vi "Proyecto Autotronicacopyy.vi"() -> ()   [LabVIEW 2026]
uses:
  <vilib>/MakerHub/LINX/Private/Type Defs/LINX Ref.ctl
  <vilib>/MakerHub/LINX/Private/Type Defs/Platform.ctl
  <vilib>/MakerHub/LINX/Private/Type Defs/Interface.ctl
  <vilib>/MakerHub/LINX/Private/Device/Type Defs/LINX Device Config.ctl
  <vilib>/MakerHub/LINX/Private/Device/Type Defs/TCP Config.ctl
  <vilib>/MakerHub/LINX/Private/Device/Type Defs/Channels.ctl
  <vilib>/MakerHub/LINX/Public/Peripherals/Digital/Digital Read 1 Chan.vi
  <vilib>/MakerHub/LINX/Public/Peripherals/Analog/Analog Read 1 Chan.vi
  <vilib>/MakerHub/LINX/Public/Peripherals/Digital/Digital Read N Chans.vi
  <vilib>/MakerHub/LINX/Public/Peripherals/Analog/Analog Read N Chans.vi
  <vilib>/MakerHub/LINX/Private/Local IO/LinxDigitalRead.vi
  <vilib>/MakerHub/LINX/Public/Utilities/Check Channel.vi
  <vilib>/MakerHub/LINX/Private/Local IO/LinxAnalogRead.vi
  <vilib>/MakerHub/LINX/Public/Utilities/Open Serial.vi
  <vilib>/MakerHub/LINX/Private/Utilties/Generate Error.vi
  <vilib>/express/express shared/transition.llb/Dynamic To Waveform Array.vi
  <vilib>/express/express signal manip/GetorSetDDTAttributes/Set DDT Attributes/SetT0.vi
  <vilib>/express/express signal manip/GetorSetDDTAttributes/Set DDT Attributes/sub Set StartTimeStamp.vi
  <vilib>/express/express shared/transition.llb/Waveform Array To Dynamic.vi
  <vilib>/express/express signal manip/GetorSetDDTAttributes/Set DDT Attributes/Set DDT Properties.xnode
  <vilib>/express/express arith-compare/Formula/XNode/ExpressFormulaBlockNode.xnode
  <vilib>/MakerHub/LINX/LMH-LINX.lvlib
  <vilib>/MakerHub/LINX/Private/Device/Device.lvlib
  <vilib>/express/express signal manip/GetorSetDDTAttributes/Set DDT Attributes/Set DDT Attributes.lvlib
panel:
  out "Waveform Chart":dbl(graph)
  out "BAR":dbl format="%#_3g"
  out "Km/hora":dbl format="%#.2g"
  out "TRAS_DER 4":bool
  out "TRAS_IZQ 3":bool
  out "DEL_IZQ":bool
  out "DEL:DER  2":bool
  out "Millas/hora":dbl format="%#.2g"
  out "Puerta 2":bool
  out "Puerta 3":bool
  out "Puerta 1":bool
  out "Llanta trasera/der":u8(slide) scale=0.0..40.0
  out "PSI":dbl format="%#_3g"
  out "BAR 2":dbl format="%#_2g"
  out "Llanta trasera/der  2":dbl(knob) scale=0.0..40.0
  out "Llanta trasera/izq":u8(slide) scale=0.0..40.0
  out "Gauge":dbl(knob) scale=0.0..200.0
  out "PSI 2":dbl format="%#_4g"
  out "BAR 3":dbl format="%#_3g"
  out "Llanta trasera/izq  2":dbl(knob) scale=0.0..40.0
  out "Llanta delantera/der":u8(slide) scale=0.0..40.0
  out "PSI 3":dbl format="%#_4g"
  out "BAR 4":dbl caption="BAR" format="%#_3g"
  out "Llanta delantera/der  2":dbl(knob) scale=0.0..40.0
  out "Llanta delantera/izq":u8(slide) scale=0.0..40.0
  out "PSI 4":dbl format="%#_4g"
  out "Llanta delantera/izq 2":dbl(knob) scale=0.0..40.0
  in  "stop":bool
  in  "Serial Port":refnum<visa-resource-name>="N/A"
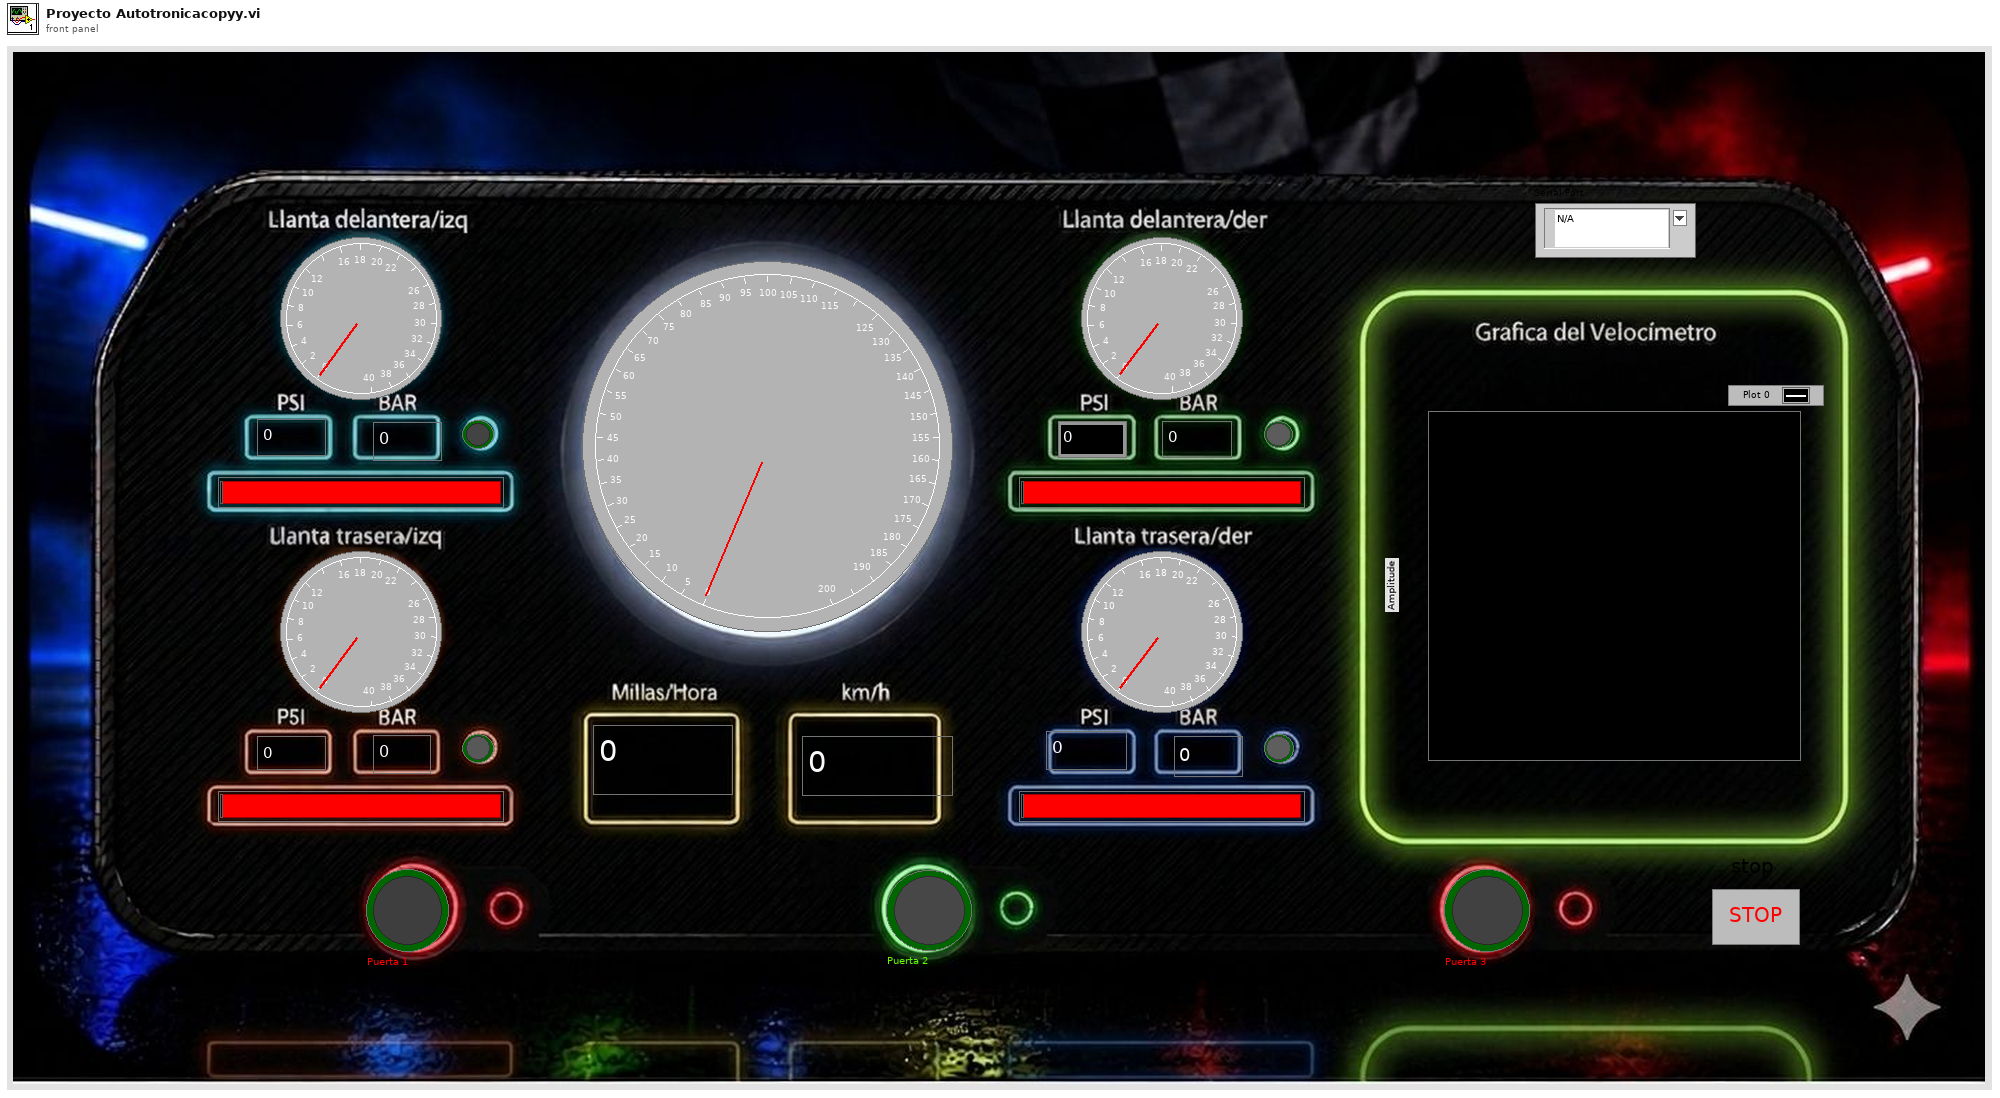
[diagram p1: front panel]
types:
  T1 = typedef "LMH-LINX.lvlib/LINX Ref.ctl" = cluster{"IO":T2, "Interface":T3, "LINX Device Config":T4}
  T2 = typedef "LMH-LINX.lvlib/Platform.ctl" = enum16{"Remote", "Local"}
  T3 = typedef "LMH-LINX.lvlib/Interface.ctl" = enum16{"Serial", "TCP"}
  T4 = typedef "LMH-LINX.lvlib/Device.lvlib/LINX Device Config.ctl" = cluster{"Interface":T3, "COM Port":refnum<visa-resource-name>, "TCP Configuration":T5, "Device Family":u8, "Device ID":u8, "Device Name":string, "TCP Ref":refnum<k5>, "Channels":T6}
  T5 = typedef "LMH-LINX.lvlib/Device.lvlib/TCP Config.ctl" = cluster{"IP Address":string, "Port":u16}
  T6 = typedef "LMH-LINX.lvlib/Channels.ctl" = cluster{"DI":u8[], "DO":u8[], "AI":u8[], "AO":u8[], "PWM":u8[], "QE":u8[], "UART":u8[], "I2C 2":u8[], "SPI":u8[], "CAN":u8[], "Servo":u8[], "AI Ref (V)":dbl, "AI Resolution (Bits)":u8, "AO Ref (V)":dbl, "AO Resolution (Bits)":u8}
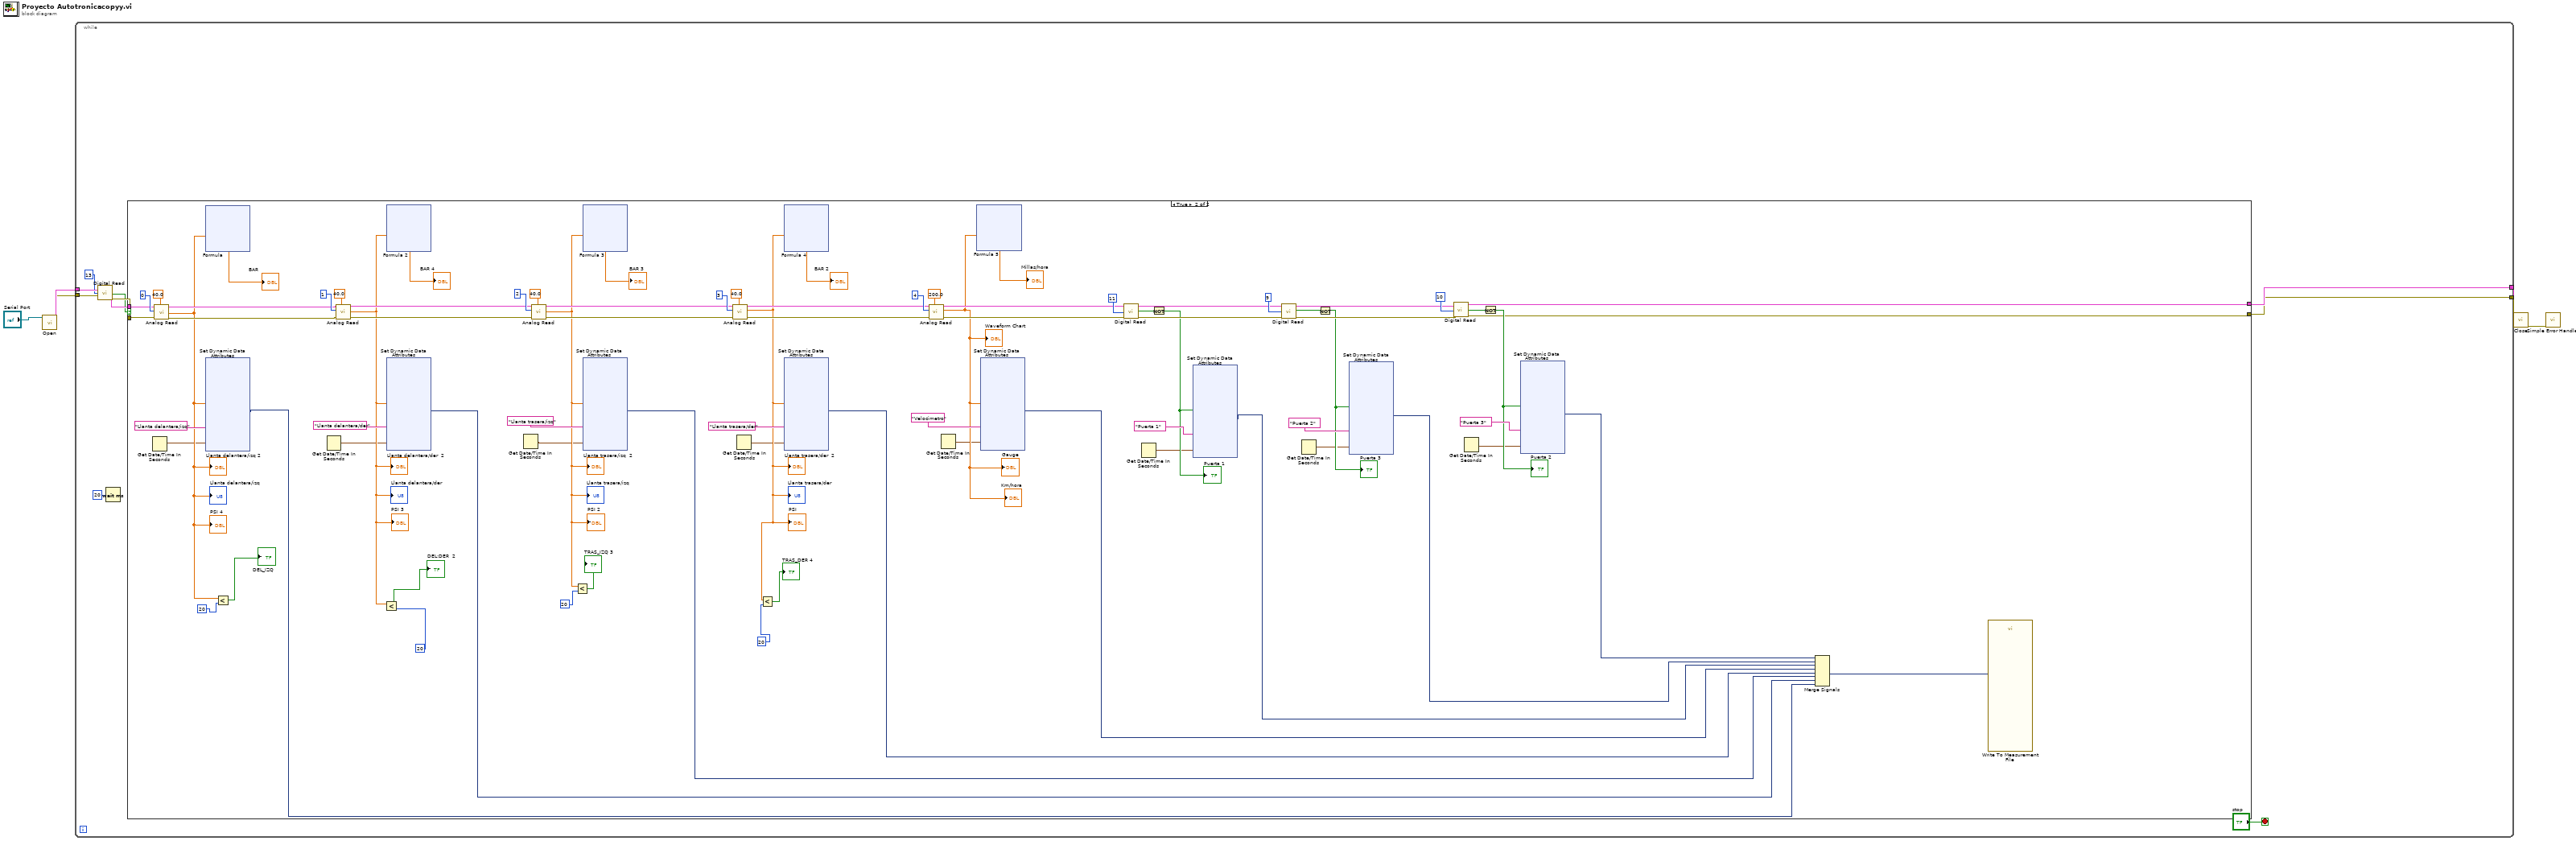
[diagram p0: block diagram]
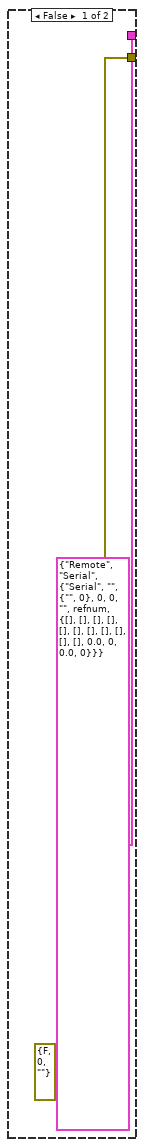
[diagram p2: hidden frame]
diagram:
  n1 = call-poly <vilib>:"Open.vi"("Serial Port"="Serial Port") -> ("Error Out"=w4:errorcluster, "LINX Resource"=w5:T1)  [unwired: 8 in, 1 out]
  n2 = while {
    tunnel: w5 -> [w16]
    tunnel: w4 -> [w15]
    tunnel: [w10] -> w1
    tunnel: [w9] -> w2
    stop <- "stop" stop-if-true
    n3 = call-poly <vilib>:"Digital Read.vi"("Error In"=w15, "DI Channel"=13, "LINX Resource"=w16) -> ("Error Out"=w12:errorcluster, "DI Value"=w7:bool, "LINX Resource"=w13:T1)  [unwired: 6 in]
    n4 = Wait (ms)(milliseconds to wait=u32 20) -> ()  [unwired: 1 out]
    n5 = case shown="True" w7 {
      tunnel: w13 -> [_ w31]
      tunnel: w12 -> [_ w30]
      tunnel: [T1 {"IO"=enum."Remote", "Interface"=enum."Serial", "LINX Device Config"={"Interface"=enum."Serial", "COM Port"="", "TCP Configuration"={"IP Address"="", "Port"=0}, "Device Family"=0, "Device ID"=0, "Device Name"="", "TCP Ref"=refnum, "Channels"={"DI"=[], "DO"=[], "AI"=[], "AO"=[], "PWM"=[], "QE"=[], "UART"=[], "I2C 2"=[], "SPI"=[], "CAN"=[], "Servo"=[], "AI Ref (V)"=0.0, "AI Resolution (Bits)"=0, "AO Ref (V)"=0.0, "AO Resolution (Bits)"=0}}} ("LINX Resource") w28] -> w10
      tunnel: [errorcluster {"status"=FALSE, "code"=0, "source"=""} ("Error Out") w29] -> w9
      frame False {
      }
      frame True {
        n6 = Get Date/Time In Seconds() -> (seconds since 1Jan1904=w19:timestamp)
        n7 = call-poly <vilib>:"Analog Read.vi"("Analog Ref Override (V)"=40.0, "Error In"=w30, "Analog Channel"=0, "LINX Resource"=w31) -> ("Error Out"=w81:errorcluster, "Voltage"=w44:dbl, "LINX Resource"=w87:T1)  [unwired: 4 in, 1 out]
        "Llanta delantera/izq 2" <- w44
        "PSI 4" <- w44
        "Llanta delantera/izq" <- w44
        n8 = xnode "Formula"("X1"=w44) -> ("Result"=→"BAR":dbl)  [unwired: 1 in, 1 out]
        n9 = xnode "Set Dynamic Data Attributes"("Signals In"=w44, "Signal Name"="Llanta delantera/izq", "Timestamp"=w19) -> ("Signals Out"=w59:dynamicdata)  [unwired: 3 in, 1 out]
        n10 = Less?(x=w44, y=20) -> (x < y?=→"DEL_IZQ":bool)
        n11 = Get Date/Time In Seconds() -> (seconds since 1Jan1904=w20:timestamp)
        n12 = call-poly <vilib>:"Analog Read.vi"("Analog Ref Override (V)"=40.0, "Error In"=w81, "Analog Channel"=1, "LINX Resource"=w87) -> ("Error Out"=w80:errorcluster, "Voltage"=w41:dbl, "LINX Resource"=w88:T1)  [unwired: 4 in, 1 out]
        "Llanta delantera/der  2" <- w41
        "PSI 3" <- w41
        "Llanta delantera/der" <- w41
        n13 = Less?(x=w41, y=20) -> (x < y?=→"DEL:DER  2":bool)
        n14 = xnode "Formula 2"("X1"=w41) -> ("Result"=→"BAR 4":dbl)  [unwired: 1 in, 1 out]
        n15 = xnode "Set Dynamic Data Attributes"("Signals In"=w41, "Signal Name"="Llanta delantera/der", "Timestamp"=w20) -> ("Signals Out"=w58:dynamicdata)  [unwired: 3 in, 1 out]
        n16 = Get Date/Time In Seconds() -> (seconds since 1Jan1904=w21:timestamp)
        n17 = call-poly <vilib>:"Analog Read.vi"("Analog Ref Override (V)"=40.0, "Error In"=w80, "Analog Channel"=2, "LINX Resource"=w88) -> ("Error Out"=w79:errorcluster, "Voltage"=w39:dbl, "LINX Resource"=w82:T1)  [unwired: 4 in, 1 out]
        "Llanta trasera/izq  2" <- w39
        "PSI 2" <- w39
        "Llanta trasera/izq" <- w39
        n18 = Less?(x=w39, y=20) -> (x < y?=→"TRAS_IZQ 3":bool)
        n19 = xnode "Formula 3"("X1"=w39) -> ("Result"=→"BAR 3":dbl)  [unwired: 1 in, 1 out]
        n20 = xnode "Set Dynamic Data Attributes"("Signals In"=w39, "Signal Name"="Llanta trasera/izq", "Timestamp"=w21) -> ("Signals Out"=w57:dynamicdata)  [unwired: 3 in, 1 out]
        n21 = call-poly <vilib>:"Analog Read.vi"("Analog Ref Override (V)"=40.0, "Error In"=w79, "Analog Channel"=3, "LINX Resource"=w82) -> ("Error Out"=w74:errorcluster, "Voltage"=w36:dbl, "LINX Resource"=w75:T1)  [unwired: 4 in, 1 out]
        "Llanta trasera/der  2" <- w36
        "PSI" <- w36
        "Llanta trasera/der" <- w36
        n22 = Get Date/Time In Seconds() -> (seconds since 1Jan1904=w22:timestamp)
        n23 = Less?(x=w36, y=20) -> (x < y?=→"TRAS_DER 4":bool)
        n24 = xnode "Formula 4"("X1"=w36) -> ("Result"=→"BAR 2":dbl)  [unwired: 1 in, 1 out]
        n25 = xnode "Set Dynamic Data Attributes"("Signals In"=w36, "Signal Name"="Llanta trasera/der", "Timestamp"=w22) -> ("Signals Out"=w56:dynamicdata)  [unwired: 3 in, 1 out]
        n26 = call-poly <vilib>:"Analog Read.vi"("Analog Ref Override (V)"=200.0, "Error In"=w74, "Analog Channel"=4, "LINX Resource"=w75) -> ("Error Out"=w67:errorcluster, "Voltage"=w27:dbl, "LINX Resource"=w71:T1)  [unwired: 4 in, 1 out]
        "Gauge" <- w27
        "Km/hora" <- w27
        "Waveform Chart" <- w27
        n27 = Get Date/Time In Seconds() -> (seconds since 1Jan1904=w23:timestamp)
        n28 = xnode "Formula 5"("X1"=w27) -> ("Result"=→"Millas/hora":dbl)  [unwired: 1 in, 1 out]
        n29 = xnode "Set Dynamic Data Attributes"("Signals In"=w27, "Signal Name"="Velocimetro", "Timestamp"=w23) -> ("Signals Out"=w55:dynamicdata)  [unwired: 3 in, 1 out]
        n30 = call-poly <vilib>:"Digital Read.vi"("Error In"=w67, "DI Channel"=11, "LINX Resource"=w71) -> ("Error Out"=w66:errorcluster, "DI Value"=w50:bool, "LINX Resource"=w69:T1)  [unwired: 6 in]
        n31 = Get Date/Time In Seconds() -> (seconds since 1Jan1904=w24:timestamp)
        n32 = Not(x=w50) -> (.not. x?=w51:bool)
        "Puerta 1" <- w51
        n33 = xnode "Set Dynamic Data Attributes"("Signals In"=w51, "Signal Name"="Puerta 1", "Timestamp"=w24) -> ("Signals Out"=w54:dynamicdata)  [unwired: 3 in, 1 out]
        n34 = call-poly <vilib>:"Digital Read.vi"("Error In"=w66, "DI Channel"=9, "LINX Resource"=w69) -> ("Error Out"=w62:errorcluster, "DI Value"=w48:bool, "LINX Resource"=w63:T1)  [unwired: 6 in]
        n35 = Get Date/Time In Seconds() -> (seconds since 1Jan1904=w26:timestamp)
        n36 = Not(x=w48) -> (.not. x?=w49:bool)
        "Puerta 3" <- w49
        n37 = xnode "Set Dynamic Data Attributes"("Signals In"=w49, "Signal Name"="Puerta 2", "Timestamp"=w26) -> ("Signals Out"=w52:dynamicdata)  [unwired: 3 in, 1 out]
        n38 = call-poly <vilib>:"Digital Read.vi"("Error In"=w62, "DI Channel"=10, "LINX Resource"=w63) -> ("Error Out"=w29:errorcluster, "DI Value"=w47:bool, "LINX Resource"=w28:T1)  [unwired: 6 in]
        n39 = Get Date/Time In Seconds() -> (seconds since 1Jan1904=w25:timestamp)
        n40 = Not(x=w47) -> (.not. x?=w46:bool)
        "Puerta 2" <- w46
        n41 = xnode "Set Dynamic Data Attributes"("Signals In"=w46, "Signal Name"="Puerta 3", "Timestamp"=w25) -> ("Signals Out"=w53:dynamicdata)  [unwired: 3 in, 1 out]
        n42 = Merge Signals(w53, w52, w54, w55, w56, w57, w58, w59) -> (w60:dynamicdata)
        n43 = call "Write To Measurement File"("Signals"=w60) -> ()  [unwired: 16 in, 3 out]
      }
    }
  }
  n44 = call <vilib>:"Close.vi"("Error In"=w2, "LINX Resource"=w1) -> ("Error Out"=w3:errorcluster)  [unwired: 9 in]
  n45 = call <vilib>:"Simple Error Handler.vi"("error in (no error)"=w3) -> ()  [unwired: 4 in, 5 out]
